vi "Initialize WORD.vi"(8 "error in (no error)":errorcluster, 11 "NI_report in":refnum<class "NI_report.lvclass">) -> (0 "error out":errorcluster, 3 "NI_report out":refnum<class "NI_report.lvclass">)   [LabVIEW 2015, in "Report.lvlib"]
uses:
  Report.lvlib
  <vilib>/Utility/NIReport.llb/NI_report.lvclass
  <vilib>/Utility/NIReport.llb/Append Report Text (str wrap).vi
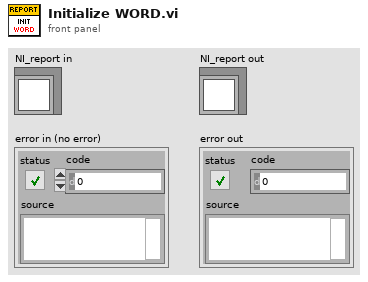
[diagram p1: front panel]
types:
  T1 = cluster{"Charset (-1)":i16, "Weight (-1)":i16, "Name":string, "Size":string}
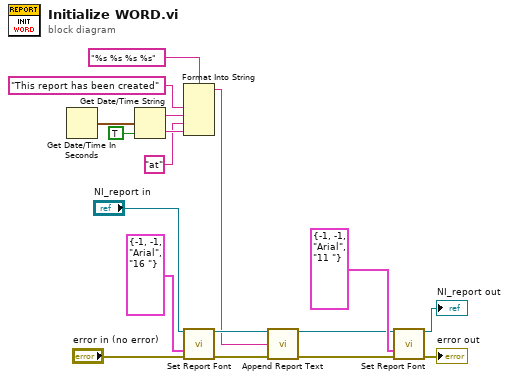
[diagram p0: block diagram]
diagram:
  n1 = Get Date/Time In Seconds() -> (seconds since 1Jan1904=w1:timestamp)
  n2 = Get Date/Time String(seconds (now)=w1, want seconds? (F)=TRUE) -> (date string=w4:string, time string=w7:string)  [unwired: 1 in]
  n3 = Format Into String(format string="%s %s %s %s", "This report has been created" ("input 1"), w4, "at" ("input 3"), w7) -> (resulting string=w8:string)  [unwired: 2 in, 1 out]
  n4 = call-dynamic "Set Report Font.vi"("report in"="NI_report in", "font settings"=T1 {"Charset (-1)"=-1, "Weight (-1)"=-1, "Name"="Arial", "Size"="16 "}, "error in (no error)"="error in (no error)") -> ("report out"=w11:refnum<class "NI_report.lvclass">, "error out"=w12:errorcluster)  [unwired: 10 in, 1 out]
  n5 = call-poly <vilib>:"Append Report Text.vi"("report in"=w11, "text"=w8, "error in (no error)"=w12) -> ("report out"=w14:refnum<class "NI_report.lvclass">, "error out"=w16:errorcluster)  [unwired: 9 in, 2 out]
  n6 = call-dynamic "Set Report Font.vi"("report in"=w14, "font settings"=T1 {"Charset (-1)"=-1, "Weight (-1)"=-1, "Name"="Arial", "Size"="11 "}, "error in (no error)"=w16) -> ("report out"=→"NI_report out":refnum<class "NI_report.lvclass">, "error out"=→"error out":errorcluster)  [unwired: 10 in, 1 out]
